vi "playWaveformAudio.vi"(5 "physical channels":tag="myDAQ1/audioOutputLeft, myDAQ1/audioOutputRight", 6 "Enum":T1=enum."Scale Audio", 7 "stop playback notifier refnum":refnum<notifier>, 8 "error in (no error)":errorcluster, 9 "sample rate (S/s)":dbl=1000.0 format="%0.2f", 10 "samples per channel":i32=1000, 11 "input waveform array":waveform(dbl)[](array[waveform])) -> (0 "error out":errorcluster)   [LabVIEW 2020]
doc: "This VI takes in an array of waveforms and outputs them on the corresponding DAQ channels. The sample clock is set to match the sampling rate of the audio, and will play the finite number of samples contained in the waveform before exiting. The VI can be aborted at any time by sending a value of True to the \"Stop Playback Notifier\""
uses:
  clipOption.ctl
  <vilib>/DAQmx/write.llb/DAQmx Write (Analog 1D Wfm NChan NSamp).vi
  <vilib>/DAQmx/create/channels.llb/DAQmx Create Channel (AO-Voltage-Basic).vi
  <vilib>/DAQmx/configure/timing.llb/DAQmx Timing (Sample Clock).vi
  <vilib>/DAQmx/miscellaneous.llb/DAQmx Fill In Error Info.vi
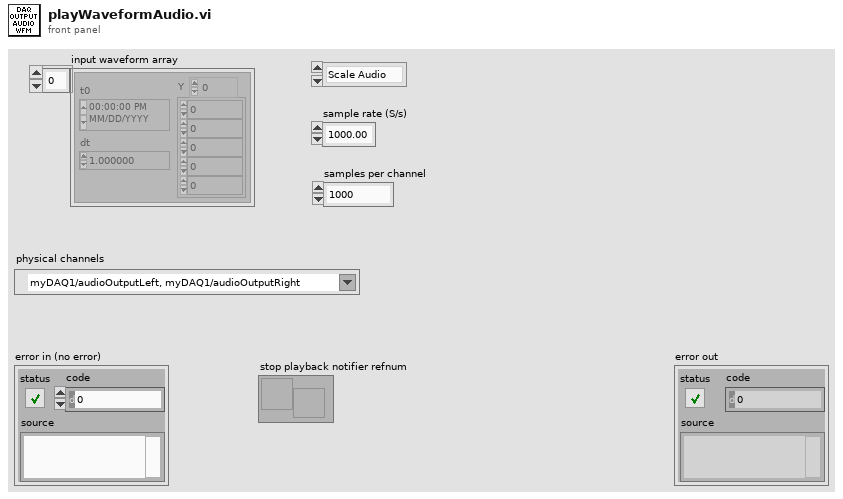
[diagram p1: front panel]
types:
  T1 = typedef "clipOption.ctl" = enum16{"Clip Audio", "Scale Audio"}
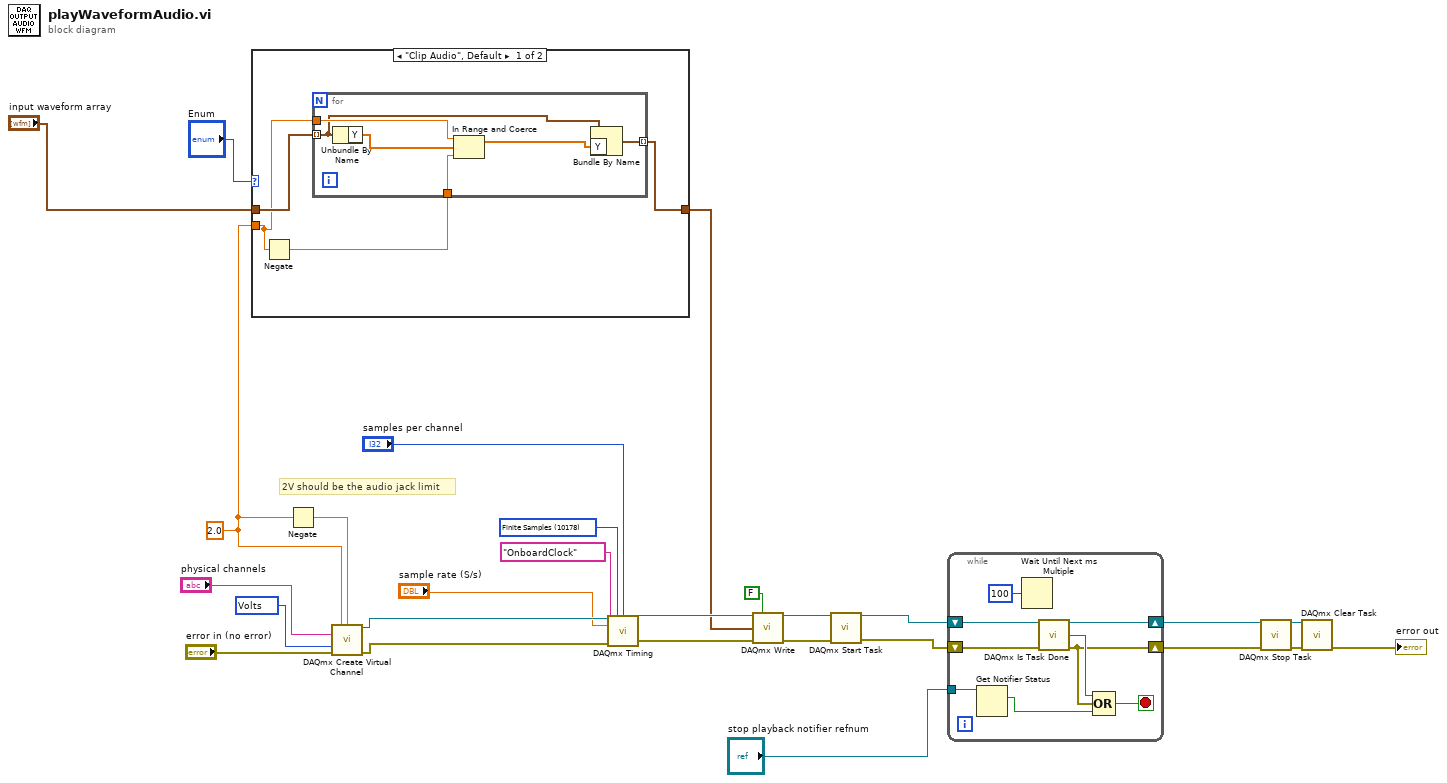
[diagram p0: block diagram]
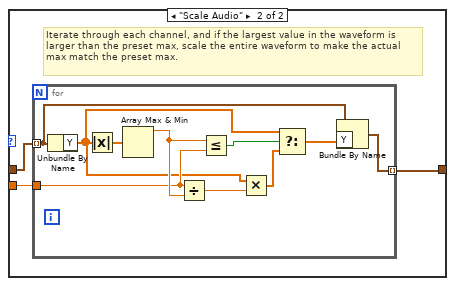
[diagram p2: hidden frame]
diagram:
  w23 = 10348 items=["Volts"=10348, "From Custom Scale"=10065] ("units")
  w1 = 2.0 ("maximum value")
  w20 = 10178 items=["Finite Samples"=10178, "Continuous Samples"=10123, "Hardware Timed Single Point"=12522] ("sample mode")
  # "2V should be the audio jack limit"
  n1 = case shown="\"Clip Audio\", Default" "Enum" {
    tunnel: "input waveform array" -> [w31 w40]
    tunnel: [w28 w38] -> w2
    tunnel: w1 -> [w29 w39]
    frame "Clip Audio", Default {
      n2 = Negate(x=w29) -> (-x=w30:dbl)
      n3 = for {
        tunnel: w31 -> [w33] mode=indexing
        tunnel: w30 -> [w36]
        tunnel: w29 -> [w35]
        tunnel: [w32] -> w28 mode=indexing
        n4 = Unbundle By Name(w33) -> ("Y"=w37:dbl[])
        n5 = In Range and Coerce(upper limit=w35, x=w37, lower limit=w36) -> (coerced(x)=w34:dbl[])  [unwired: 1 out]
        n6 = Bundle By Name(cluster=w33, "Y"=w34) -> (w32:waveform(dbl))
      }
    }
    frame "Scale Audio" {
      # "Iterate through each channel, and if the largest value in the waveform is larger than the preset max, scale the entire waveform to make the actual max match the preset max."
      n7 = for {
        tunnel: w40 -> [w43] mode=indexing
        tunnel: w39 -> [w47]
        tunnel: [w41] -> w38 mode=indexing
        n8 = Unbundle By Name(w43) -> ("Y"=w45:dbl[])
        n9 = Absolute Value(x=w45) -> (abs(x)=w50:dbl[])
        n10 = Array Max & Min(array=w50) -> (max value=w48:dbl)  [unwired: 3 out]
        n11 = Divide(x=w47, y=w48) -> (x/y=w49:dbl)
        n12 = Less Or Equal?(x=w48, y=w47) -> (x <= y?=w46:bool)
        n13 = Multiply(x=w45, y=w49) -> (x*y=w44:dbl[])
        n14 = Select(t=w45, s=w46, f=w44) -> (s? t:f=w42:dbl[])
        n15 = Bundle By Name(cluster=w43, "Y"=w42) -> (w41:waveform(dbl))
      }
    }
  }
  n16 = Negate(x=w1) -> (-x=w22:dbl)
  n17 = call-poly <vilib>:"DAQmx Create Virtual Channel.vi"("maximum value"=w1, "minimum value"=w22, "physical channels"="physical channels", "units"=w23, "error in"="error in (no error)") -> ("task out"=w16:refnum<k21>, "error out"=w19:errorcluster)  [unwired: 9 in]
  n18 = call-poly <vilib>:"DAQmx Timing.vi"("task/channels in"=w16, "sample mode"=w20, "samples per channel"="samples per channel", "rate"="sample rate (S/s)", "source"=tag "OnboardClock", "error in"=w19) -> ("task out"=w17:refnum<k21>, "error out"=w18:errorcluster)  [unwired: 8 in]
  n19 = call-poly <vilib>:"DAQmx Write.vi"("task/channels in"=w17, "auto start"=FALSE, "data"=w2, "error in"=w18) -> ("task out"=w14:refnum<k21>, "error out"=w15:errorcluster)  [unwired: 9 in, 1 out]
  n20 = call <vilib>:"DAQmx Start Task.vi"("task/channels in"=w14, "error in"=w15) -> ("task out"=w25:refnum<k21>, "error out"=w26:errorcluster)  [unwired: 12 in]
  n21 = while {
    shift-right: [w58] -> w9
    shift-left: w25 -> [w59]
    shift-right: [w55] -> w8
    shift-left: w26 -> [w57]
    tunnel: "stop playback notifier refnum" -> [w52]
    stop <- w54 stop-if-true
    n22 = Get Notifier Status(notifier=w52) -> (current notification=w51:bool)  [unwired: 1 in, 4 out]
    n23 = Wait Until Next ms Multiple(millisecond multiple=u32 100) -> ()  [unwired: 1 out]
    n24 = call <vilib>:"DAQmx Is Task Done.vi"("task/channels in"=w59, "error in"=w57) -> ("task out"=w58:refnum<k21>, "task done?"=w56:bool, "error out"=w55:errorcluster)  [unwired: 11 in]
    n25 = Compound Arithmetic op=OR(w56, w55, w51) -> (w54:bool)
  }
  n26 = call <vilib>:"DAQmx Stop Task.vi"("task/channels in"=w9, "error in"=w8) -> ("task out"=w11:refnum<k21>, "error out"=w10:errorcluster)  [unwired: 12 in]
  n27 = call <vilib>:"DAQmx Clear Task.vi"("task in"=w11, "error in"=w10) -> ("error out"=→"error out":errorcluster)  [unwired: 13 in]
